vi "Response.vi"(8 "error in (no error)":errorcluster, 11 "JSON Value in":refnum<class "JSON Value.lvclass">) -> (0 "error out":errorcluster, 2 "values":string[](array[string]), 3 "keys":string[](array[string]))   [LabVIEW 2021]
uses:
  <vilib>/NI/JSON Support for LabVIEW/JSON Value/JSON Value.lvclass
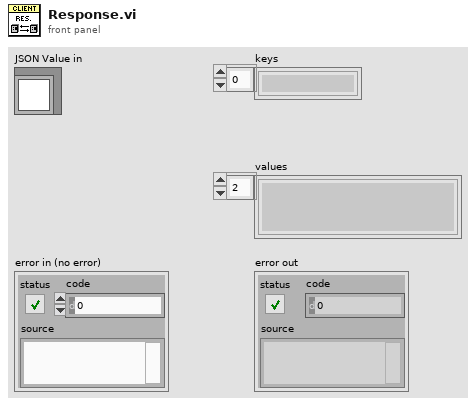
[diagram p1: front panel]
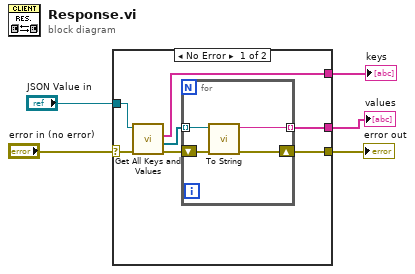
[diagram p0: block diagram]
diagram:
  n1 = case shown="No Error" "error in (no error)" {
    selector: "error in (no error)" -> [w12 w17]
    tunnel: "JSON Value in" -> [w6 _]
    tunnel: [w10 w17] -> w1
    tunnel: [w9 _] -> w2
    tunnel: [w8 _] -> w3
    frame No Error {
      n2 = call <vilib>:"Get All Keys and Values.vi"("error in"=w12, "JSON Value in"=w6) -> ("error out"=w11:errorcluster, "values"=w7:refnum<class "JSON Value.lvclass">[], "keys"=w8:string[])  [unwired: 7 in]
      n3 = for {
        tunnel: w7 -> [w15] mode=indexing
        shift-right: [w14] -> w10
        shift-left: w11 -> [w16]
        tunnel: [w13] -> w9 mode=indexing
        n4 = call <vilib>:"To String.vi"("error in (no error)"=w16, "JSON Value in"=w15) -> ("error out"=w14:errorcluster, "String"=w13:string)  [unwired: 8 in]
      }
    }
    frame Error {
    }
  }
  "keys" <- w3
  "values" <- w2
  "error out" <- w1
